vi "PFI-28000-Utils_Wait.vi"(0 "Time (ms)":u32, 11 "error in (no error)":errorcluster) -> (4 "Timer Value":u32, 15 "error out":errorcluster)   [LabVIEW 2017, in "PFI-28000-Utils.lvlib"]
uses:
  PFI-28000-Utils.lvlib
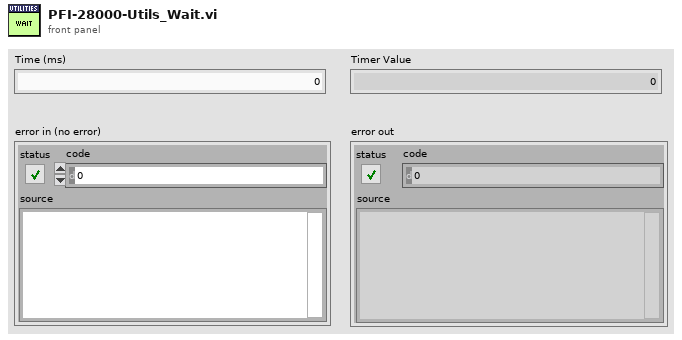
[diagram p1: front panel]
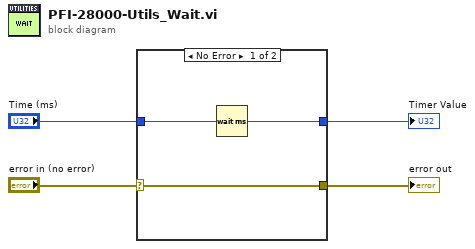
[diagram p0: block diagram]
diagram:
  n1 = case shown="No Error" "error in (no error)" {
    selector: "error in (no error)" -> [w5 w8]
    tunnel: "Time (ms)" -> [w7 _]
    tunnel: [w6 _] -> w3
    tunnel: [w5 w8] -> w1
    frame No Error {
      n2 = Wait (ms)(milliseconds to wait=w7) -> (millisecond timer value=w6:u32)
    }
    frame Error {
    }
  }
  "error out" <- w1
  "Timer Value" <- w3
